vi "Beam_Max_Pos.vi"(1 "Picture Log":path, 5 "Search Step (mm)":dbl=1.0, 6 "Mode":T6, 7 "Starting Position":dbl[](array[numeric]) format="%.1f", 8 "Traverse line In":T1 {"Carrier_2 Q (l/min)" format="%#.2f"; "Row Duration (mins)" format="%#.1f"; "Row No" min=0; "Trace Gas Concentration (%)" min=0.0 format="%#_4f"; "Carrier_1 Q (l/min)" format="%#.2f"; "Tunnel Speed" format="%#.2f"; "Start X" format="%#.2f"; "Start Y" format="%#.2f"; "Start Z" format="%#.2f"; "End X" format="%#.2f"; "End Y" format="%#.2f"; "End Z" format="%#.2f"; "Averaging time (min)" min=0.0 format="%#.2f"}, 9 "Fixed Axis":T4, 10 "Beam Name":string) -> (0 "Power at Maxima":dbl, 2 "Status":T5, 3 "Beam maxima":dbl[](array[numeric]) format="%.1f", 4 "Message":string)   [LabVIEW 2016]
uses:
  Controls/User_Specific_mode.ctl
  Gen Trav/Multi_Run_Status.ctl
  Gen Trav/Route mapping/Axis.ctl
  Gen Trav/Traverse_cluster.ctl
  Gen Trav/Spacing.ctl
  Controls/Multi_run_mode.ctl
panel:
  out "Server copy Location":path
  out "vi reference":refnum<vi>
  in  "stop":bool
  out "Y":i32
  out "X":i32
  out "Array 2":dbl[](array[numeric]) format="%.4f"
  out "Measured Points":dbl[][](array[numeric]) format="%.2f"
  out "Current Value":dbl format="%.2f"
  out "Current Index":i32
  out "Array":i32[][](array[numeric])
  out "Light Power Measurement":dbl[][](graph)
  out "Found Maxima?":bool
  out "Present Position":dbl[](array[numeric])
  out "Profile":dbl[][](array[numeric]) format="%.2f"
  out "Log File":path
  # "X           Y            Z"
  # "Start"
  # "End"
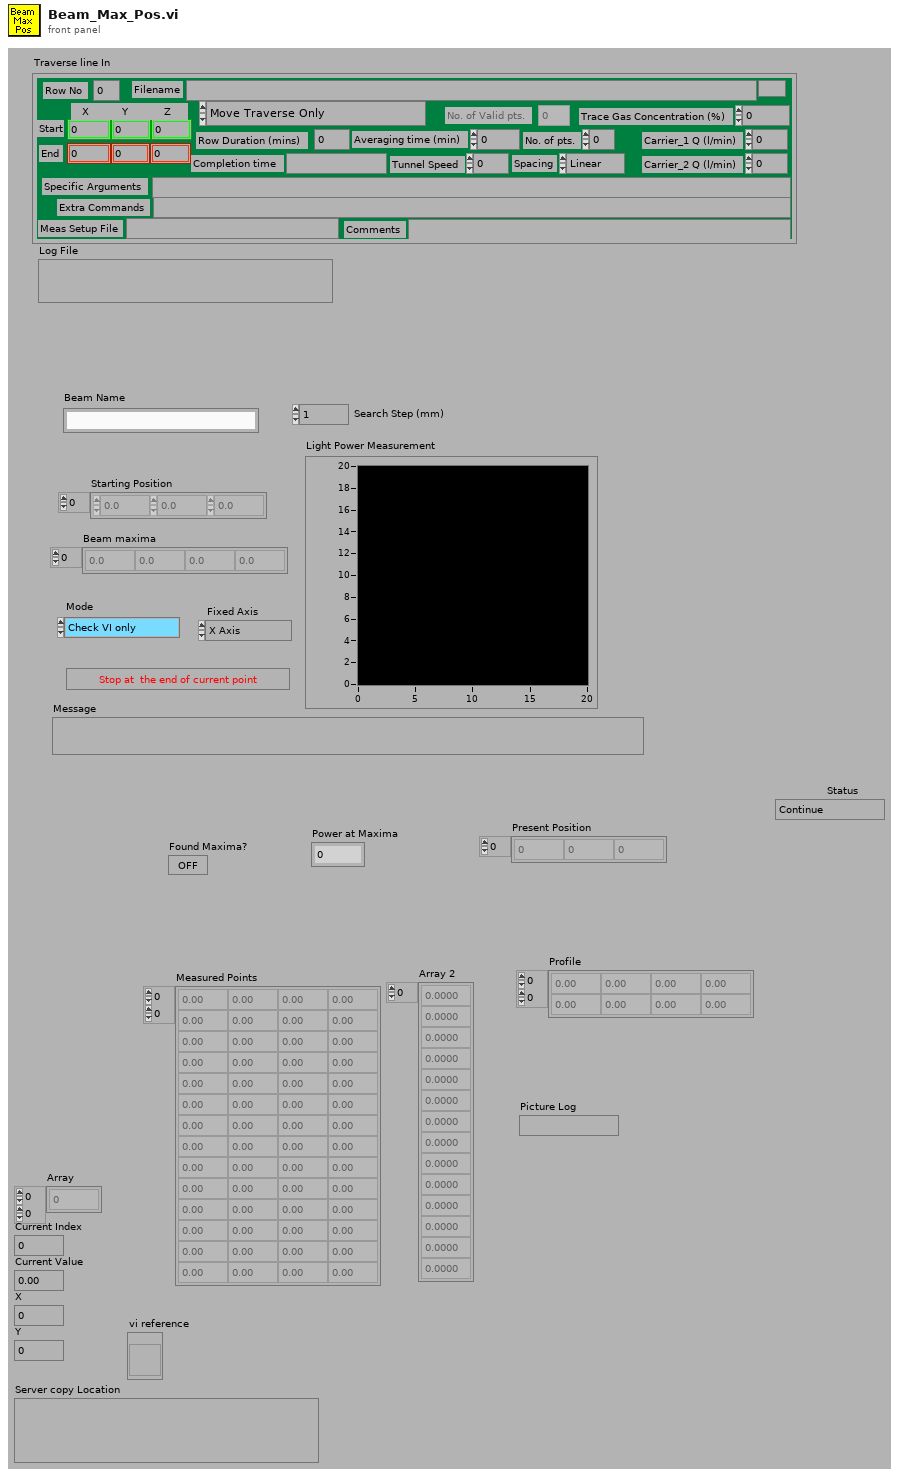
[diagram p1: front panel]
types:
  T1 = typedef "Traverse_cluster.ctl" = cluster{"Start X":sgl, "Start Y":sgl, "Start Z":sgl, "End X":sgl, "End Y":sgl, "End Z":sgl, "No. of pts.":i32, "Spacing":T2, "Filename":path, "Tunnel Speed":dbl, "Averaging time (min)":dbl, "Extra Commands":string, "Carrier_1 Q (l/min)":dbl, "Carrier_2 Q (l/min)":dbl, "Trace Gas Concentration (%)":dbl, "Specific Arguments":string, "Comments":string, "Row No":i32, "Row Type Selector":T3, "Completion time":string, "Row Duration (mins)":dbl, "No. of Valid pts.":i32, "Meas Setup File":string}
  T2 = typedef "Spacing.ctl" = enum16{"Linear", "Log", "Gauss", "Specified", "N/A"}
  T3 = typedef "Multi_run_mode.ctl" = enum16{"Move Traverse Only", "Set Tunnel Speed Only", "Set Source Only", "Set Measurement Conditions", "Single Measurement", "Vertical Profile", "Lateral Profile", "Longitudinal Profile", "Explore Volume", "Multi-Axis Profile", "Auto Calibrate", "Meas Fast FID Bkgnd", "Check Beam Power", "Scanning Valve Measurement", "Run VI Named:", "Set ADAM Ch", "Wait (minutes)", "Send Message", "Synchronize With:", "Fall Back to this Row", "Turn Off Row Repeating", "Blank Row", "Traverse 3D Volume"}
  T4 = typedef "Axis.ctl" = enum16{"X Axis", "X Axis -ve", "Y Axis", "Y Axis -ve", "Z Axis", "Z Axis -ve"}
  T5 = typedef "Multi_Run_Status.ctl" = enum16{"Continue", "Jump to Next Point", "Jump to Next Row", "Jump To Fall Back", "Terminate Run"}
  T6 = typedef "User_Specific_mode.ctl" = enum16{"Check VI only", "Run VI"}
  T7 = cluster{"Status":enum16{"Continue", "Jump to Next Point", "Jump to Next Row", "Jump To Fall Back", "Terminate Run"}, "Error Type":string, "Error Description":string}
  T8 = typedef "Status_Cluster.ctl" = cluster{"Status":T5, "Error Type":string, "Error Description":string}
  T9 = cluster{"second":i32, "minute":i32, "hour":i32, "day of month":i32, "month":i32, "year":i32, "day of week":i32, "day of year":i32, "is DST":i32}
  T10 = typedef "LVRectTypeDef.ctl" = cluster{"left":i16, "top":i16, "right":i16, "bottom":i16}
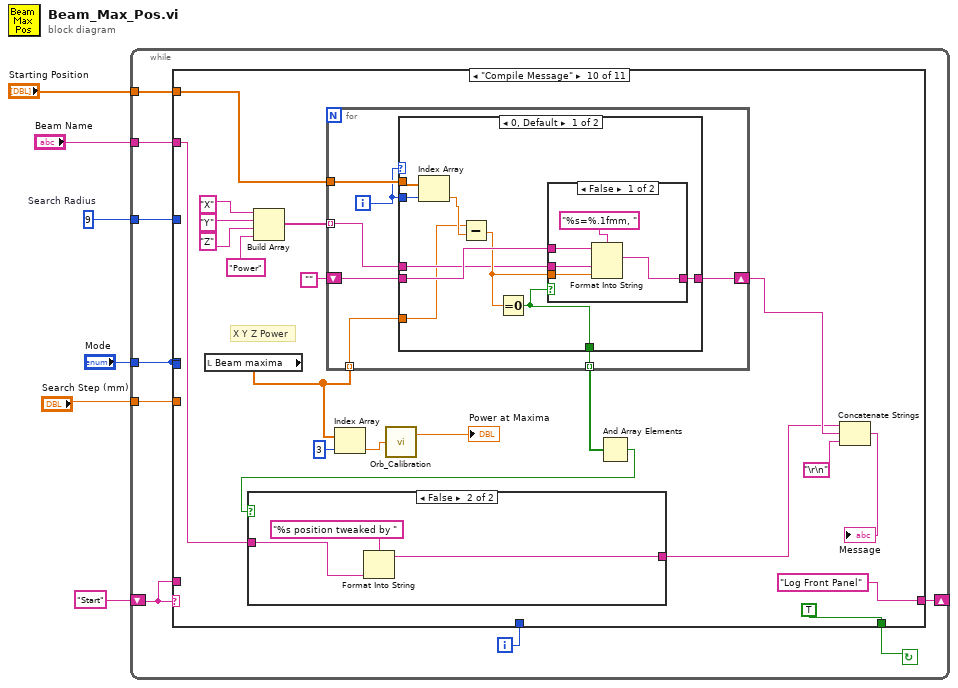
[diagram p0: block diagram]
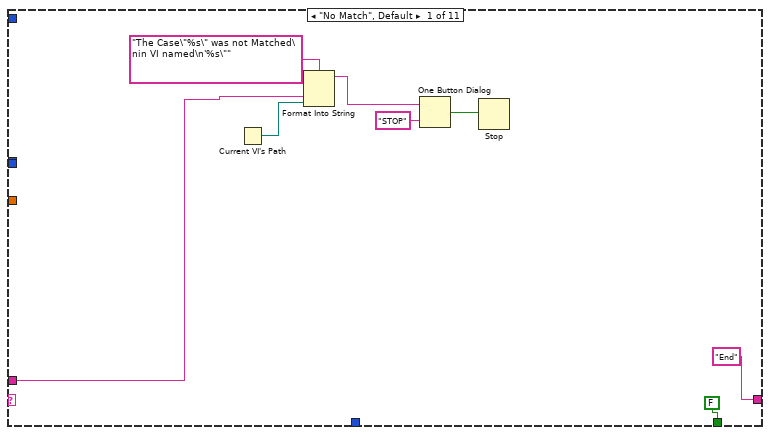
[diagram p2: hidden frame]
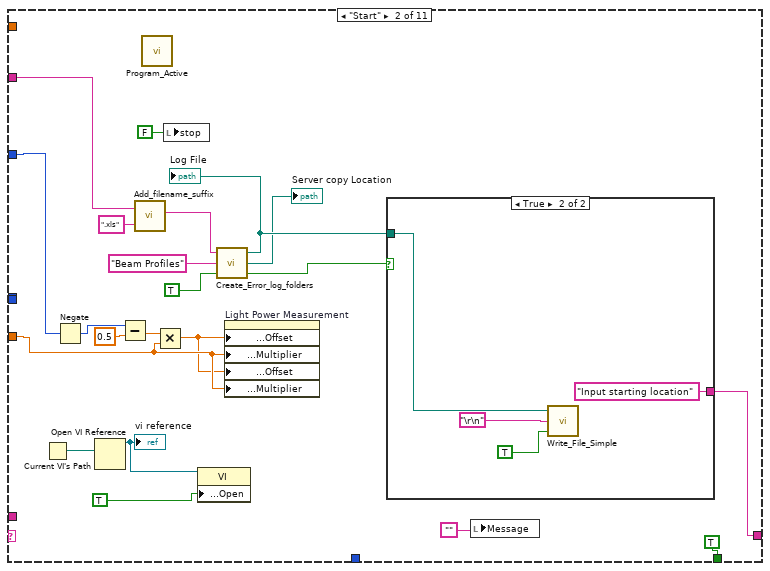
[diagram p3: hidden frame]
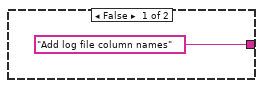
[diagram p4: hidden frame]
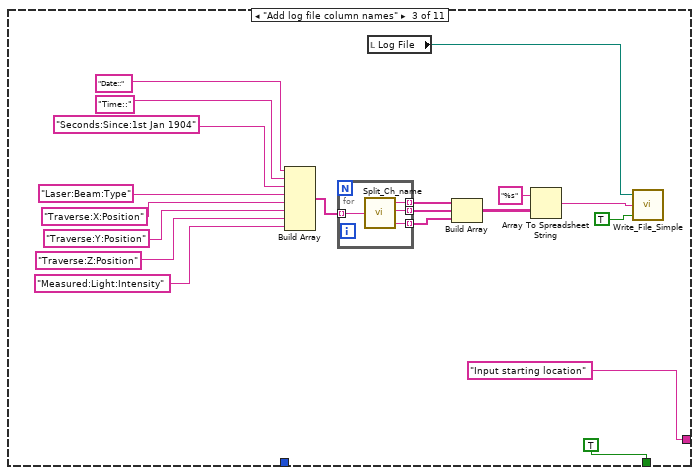
[diagram p5: hidden frame]
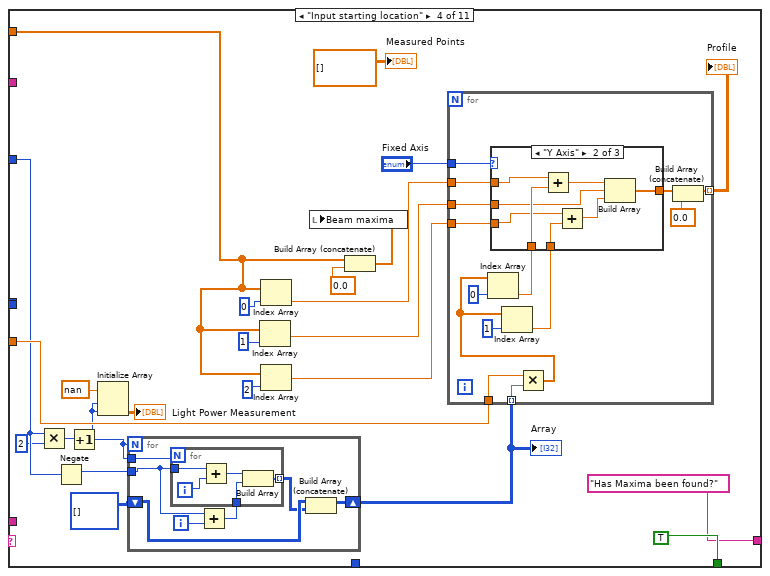
[diagram p6: hidden frame]
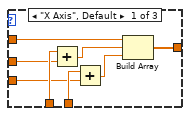
[diagram p7: hidden frame]
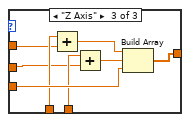
[diagram p8: hidden frame]
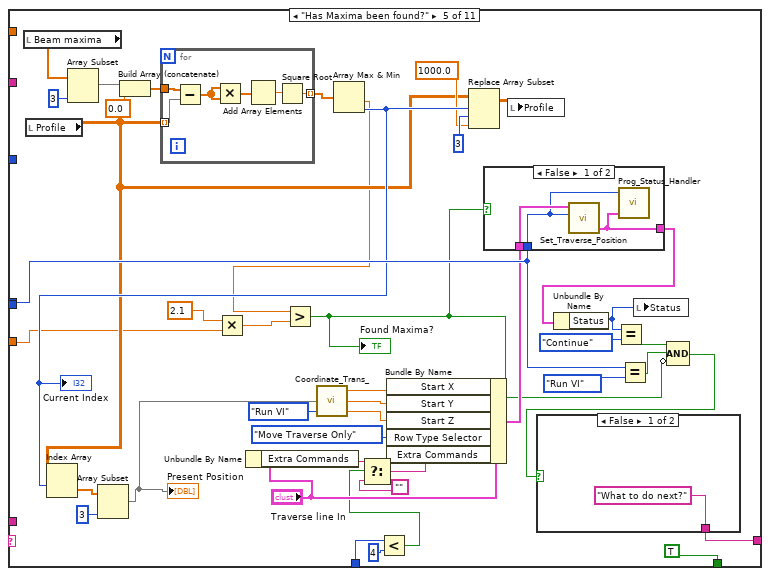
[diagram p9: hidden frame]
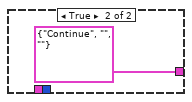
[diagram p10: hidden frame]
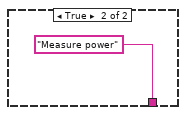
[diagram p11: hidden frame]
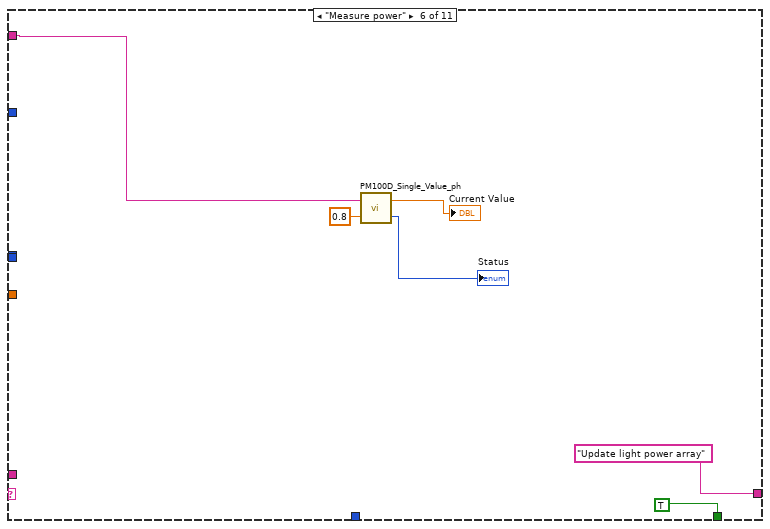
[diagram p12: hidden frame]
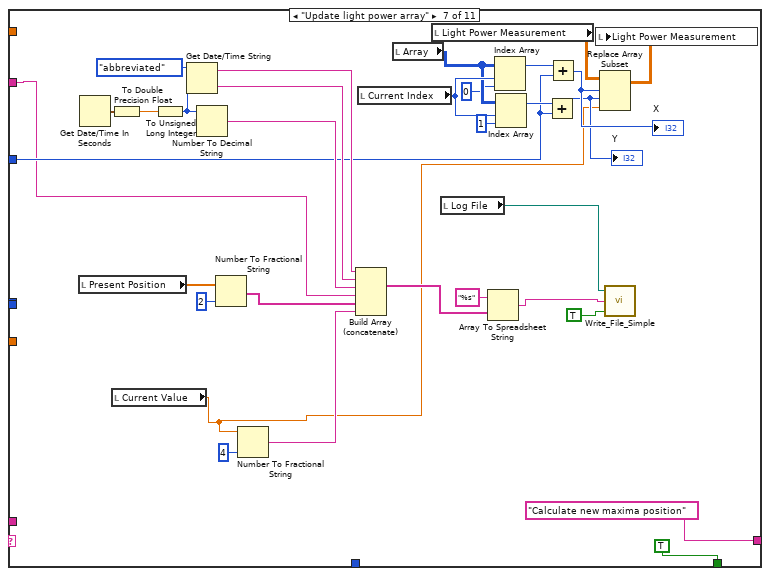
[diagram p13: hidden frame]
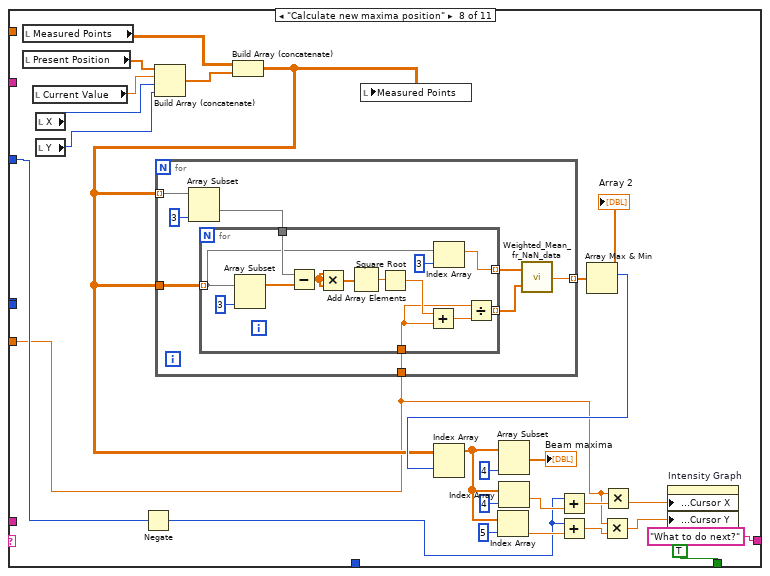
[diagram p14: hidden frame]
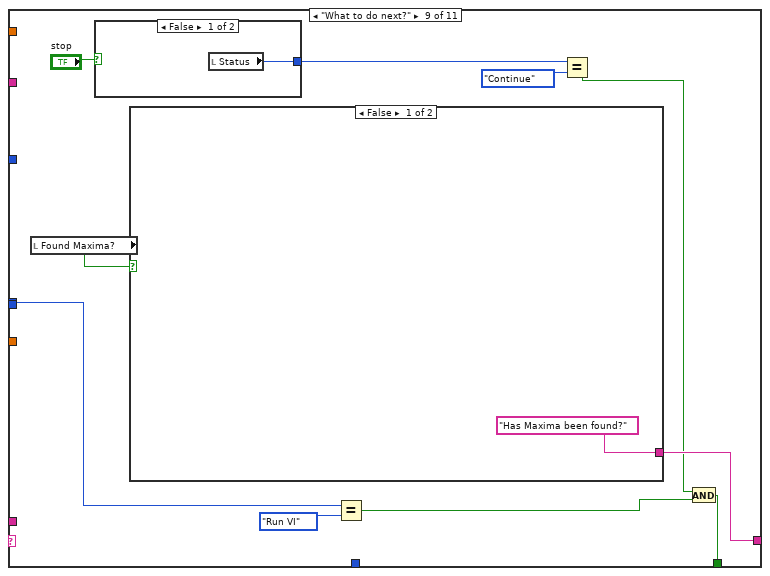
[diagram p15: hidden frame]
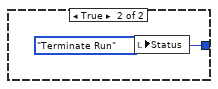
[diagram p16: hidden frame]
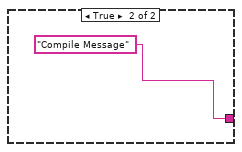
[diagram p17: hidden frame]
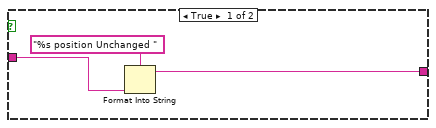
[diagram p18: hidden frame]
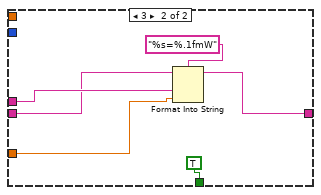
[diagram p20: hidden frame]
diagram:
  w5 = 9  # Search Radius
  n1 = while {
    tunnel: "Search Step (mm)" -> [w12]
    tunnel: "Mode" -> [w13]
    shift-left: "Start" -> [w7]
    shift-right: [w14] -> _
    tunnel: w5 -> [w11]
    tunnel: "Beam Name" -> [w10]
    tunnel: "Starting Position" -> [w9]
    i -> [w8]
    stop <- w15 continue-if-true
    n2 = case shown="\"Compile Message\"" w7 {
      tunnel: w13 -> [_ _ _ _ w184 _ _ _ w291 _ _]
      tunnel: [FALSE TRUE TRUE TRUE TRUE TRUE TRUE TRUE w285 TRUE FALSE] -> w15
      tunnel: ["End" w34 "Input starting location" "Has Maxima been found?" w163 "Update light power array" "Calculate new maxima position" "What to do next?" w288 "Log Front Panel" "End"] -> w14
      tunnel: w13 -> [_ _ _ _ _ _ _ _ _ _ _]
      tunnel: w12 -> [_ w33 _ w89 w165 _ _ w242 _ _ _]
      tunnel: w11 -> [_ w39 _ w81 _ _ w213 w246 _ _ _]
      tunnel: w10 -> [_ w37 _ _ _ w202 w211 _ _ w309 w359]
      tunnel: w9 -> [_ _ _ w74 _ _ _ _ _ w308 _]
      tunnel: w8 -> [_ _ _ _ w148 _ _ _ _ _ _]
      tunnel: w7 -> [w18 _ _ _ _ _ _ _ _ _ _]
      frame "No Match", Default {
        n3 = Current VI's Path() -> (path=w23:path)
        n4 = Format Into String(format string="The Case\"%s\" was not Matched\nin VI named\n'%s\"" ("Format String"), w18, w23) -> (resulting string=w20:string)  [unwired: 2 in, 1 out]
        n5 = One Button Dialog(message=w20, button name ("OK")="STOP") -> (true=w22:bool)
        n6 = Stop(stop? (T)=w22) -> ()
      }
      frame "Start" {
        n7 = Current VI's Path() -> (path=w28:path)
        n8 = Negate(x=w39) -> (-x=w30:i32)
        n9 = Open VI Reference(vi path=w28) -> (vi reference=w27:refnum<vi>)  [unwired: 1 in, 5 out]
        "vi reference" <- w27
        n10 = Subtract(x=w30, y=0.5) -> (x-y=w31:dbl)
        n11 = call "Add_filename_suffix.vi"("Filename"=w37, "Suffix to add"=".xls") -> ("Filename out"=w35:string)  [unwired: 3 out]
        n12 = call "Program_Active.vi"() -> ()  [unwired: 1 in]
        n13 = Multiply(x=w31, y=w33) -> (x*y=w32:dbl)
        n14 = local write "stop"(FALSE ("stop")) -> ()
        n15 = property class="VI"(reference=w27, "Front Panel Window:Open"=TRUE) -> ()  [unwired: 1 in, 2 out]
        n16 = call "Create_Error_log_folders.vi"("Per Day Log File?"=TRUE, "Log Folder"="Beam Profiles" ("Input Element"), "Log Filename"=w35) -> ("exists?"=w42:bool, "Server copy Location"=→"Server copy Location":path, "Local Log File"=w43:path)
        "Log File" <- w43
        n17 = property on="Light Power Measurement" class="IntGraph (strict)"("X Scale.Offset and Multiplier:Offset"=w32, "X Scale.Offset and Multiplier:Multiplier"=w33, "Y Scale.Offset and Multiplier:Offset"=w32, "Y Scale.Offset and Multiplier:Multiplier"=w33) -> ()  [unwired: 2 in, 2 out]
        n18 = case shown="True" w42 {
          tunnel: w43 -> [_ w46]
          tunnel: ["Add log file column names" "Input starting location"] -> w34
          frame False {
          }
          frame True {
            n19 = call "Write_File_Simple.vi"("append to file? (new file:F)"=TRUE, "character string"="\r\n", "file path"=w46) -> ()  [unwired: 2 out]
          }
        }
        n20 = local write "Message"("") -> ()
      }
      frame "Add log file column names" {
        n21 = Build Array("Date::", "Time::", "Seconds:Since:1st Jan 1904", "Laser:Beam:Type", "Traverse:X:Position", "Traverse:Y:Position", "Traverse:Z:Position", "Measured:Light:Intensity") -> (w62:string[])
        n22 = for {
          tunnel: w62 -> [w72] mode=indexing
          tunnel: [w71] -> w63 mode=indexing
          tunnel: [w70] -> w64 mode=indexing
          tunnel: [w69] -> w65 mode=indexing
          n23 = call "Split_Ch_name.vi"("Ch name"=w72) -> ("Top level"=w71:string, "Middle"=w70:string, "Low level"=w69:string)
        }
        n24 = local read "Log File"() -> (w50:path)
        n25 = Build Array(w63, w64, w65) -> (w60:string[][])
        n26 = Array To Spreadsheet String(array=w60, 3:"%s" ("format string")) -> (spreadsheet string=w51:string)  [unwired: 1 out]
        n27 = call "Write_File_Simple.vi"("append to file? (new file:F)"=TRUE, "character string"=w51, "file path"=w50) -> ()  [unwired: 2 out]
      }
      frame "Input starting location" {
        n28 = Multiply(x=w81, y=2) -> (x*y=w79:i32)
        n29 = Negate(x=w81) -> (-x=w82:i32)
        n30 = Increment(x=w79) -> (x+1=w78:i32)
        n31 = Initialize Array(nan, w78, w78) -> (→"Light Power Measurement":dbl[][])
        n32 = for {
          N: w78 -> [_]
          tunnel: w78 -> [w103]
          tunnel: w82 -> [w101]
          shift-right: [w97] -> w87
          shift-left: i32[][] [] -> [w99]
          i -> [w102]
          n33 = Add(x=w101, y=w102) -> (x+y=w100:i32)
          n34 = for {
            N: w103 -> [_]
            tunnel: w101 -> [w107]
            tunnel: w100 -> [w105]
            tunnel: [w104] -> w98 mode=indexing
            i -> [w108]
            n35 = Add(x=w107, y=w108) -> (x+y=w106:i32)
            n36 = Build Array(w106, w105) -> (w104:i32[])
          }
          n37 = Build Array (concatenate)(w99, w98) -> (w97:i32[][])
        }
        "Array" <- w87
        n38 = Index Array(array=w74, index=1 ("Index")) -> (element=w93:dbl)
        n39 = Index Array(array=w74, index=0 ("Index")) -> (element=w94:dbl)
        n40 = Index Array(array=w74, index=2 ("Index")) -> (element=w92:dbl)
        n41 = Build Array (concatenate)(w74, 0.0 ("Numeric")) -> (w90:dbl[])
        n42 = local write "Beam maxima"(w90) -> ()
        n43 = for {
          tunnel: w89 -> [w122]
          tunnel: w87 -> [w121] mode=indexing
          tunnel: "Fixed Axis" -> [w120]
          tunnel: w94 -> [w116]
          tunnel: w93 -> [w113]
          tunnel: w92 -> [w112]
          tunnel: [w110] -> w95 mode=indexing
          n44 = Multiply(x=w122, y=w121) -> (x*y=w117:dbl[])
          n45 = Index Array(array=w117, index=0 ("Index")) -> (element=w115:dbl)
          n46 = Index Array(array=w117, index=1 ("Index")) -> (element=w114:dbl)
          n47 = case shown="\"Y Axis\"" w120 {
            tunnel: w116 -> [w130 w137 w141]
            tunnel: w115 -> [w129 w135 w144]
            tunnel: w114 -> [w128 w134 w143]
            tunnel: w113 -> [w127 w131 w142]
            tunnel: w112 -> [w126 w133 w145]
            tunnel: [w123 w138 w146] -> w111
            frame "X Axis", Default {
              n48 = Add(x=w129, y=w127) -> (x+y=w125:dbl)
              n49 = Add(x=w128, y=w126) -> (x+y=w124:dbl)
              n50 = Build Array(w130, w125, w124) -> (w123:dbl[])
            }
            frame "Y Axis" {
              n51 = Add(x=w137, y=w135) -> (x+y=w136:dbl)
              n52 = Add(x=w133, y=w134) -> (x+y=w132:dbl)
              n53 = Build Array(w136, w131, w132) -> (w138:dbl[])
            }
            frame "Z Axis" {
              n54 = Add(x=w144, y=w141) -> (x+y=w140:dbl)
              n55 = Add(x=w143, y=w142) -> (x+y=w139:dbl)
              n56 = Build Array(w140, w139, w145) -> (w146:dbl[])
            }
          }
          n57 = Build Array (concatenate)(w111, 0.0 ("Input Element")) -> (w110:dbl[])
        }
        "Profile" <- w95
        "Measured Points" <- dbl[][] [] ("Measured Points")
      }
      frame "Has Maxima been found?" {
        n58 = local read "Beam maxima"() -> (w181:dbl[])
        n59 = local read "Profile"() -> (w171:dbl[][])
        n60 = Array Subset(array=w181, length=3 ("Array Length")) -> (w178:dbl[])  [unwired: 1 in]
        n61 = Build Array (concatenate)(w178, 0.0 ("Input Element")) -> (w177:dbl[])
        n62 = for {
          tunnel: w171 -> [w200] mode=indexing
          tunnel: w177 -> [w199]
          tunnel: [w195] -> w179 mode=indexing
          n63 = Subtract(x=w199, y=w200) -> (x-y=w197:dbl[])
          n64 = Multiply(x=w197, y=w197) -> (x*y=w196:dbl[])
          n65 = Add Array Elements(numeric array=w196) -> (sum=w198:dbl)
          n66 = Square Root(x=w198) -> (sqrt(x)=w195:dbl)
        }
        n67 = Multiply(x=2.1, y=w165) -> (x*y=w168:dbl)
        n68 = Unbundle By Name("Traverse line In") -> ("Extra Commands"=w160:string)
        n69 = Array Max & Min(array=w179) -> (min value=w169:dbl, min index (indices)=w175:i32)  [unwired: 2 out]
        "Current Index" <- w175
        n70 = Index Array(array=w171, index (row)=w175) -> (element=w151:dbl[])  [unwired: 1 in]
        n71 = Array Subset(array=w151, length=3) -> (w150:dbl[])  [unwired: 1 in]
        "Present Position" <- w150
        n72 = Greater?(x=w169, y=w168) -> (0:w155:bool)
        "Found Maxima?" <- w155
        n73 = call "Coordinate_Trans_.vi"("Simulate/Run"=User_Specific_mode."Run VI", "Input Position"=w150) -> ("Z"=w154:sgl, "Y"=w153:sgl, "X"=w152:sgl)  [unwired: 1 in]
        n74 = Less?(x=w148, y=4) -> (x < y?=w158:bool)
        n75 = Select(t=w160, s=w158, f="") -> (s? t:f=w156:string)
        n76 = Bundle By Name(cluster="Traverse line In", "Start X"=w152, "Start Y"=w153, "Start Z"=w154, "Row Type Selector"=Multi_run_mode."Move Traverse Only", "Extra Commands"=w156) -> (w164:T1)
        n77 = Replace Array Subset(array=w171, new element=1000.0 ("Element Data"), index (row)=w175, index (col)=3 ("Index")) -> (w172:dbl[][])
        n78 = case shown="False" w155 {
          tunnel: [w190 T7 {"Status"=enum."Continue", "Error Type"="", "Error Description"=""} ("Status Cluster")] -> w186
          tunnel: w184 -> [w189 _]
          tunnel: w164 -> [w191 _]
          frame False {
            n79 = call "Set_Traverse_Position.vi"("Simulate/Run"=w189, "Traverse line"=w191) -> ("Status Cluster"=w190:T8)  [unwired: 4 in]
            n80 = call "Prog_Status_Handler.vi"("Status Cluster"=w190, "Simulate/Run"=w189) -> ()  [unwired: 2 out]
          }
          frame True {
          }
        }
        n81 = local write "Profile"(w172) -> ()
        n82 = Unbundle By Name(w186) -> ("Status"=w182:T5)
        n83 = Equal?(x=w182, y=Multi_Run_Status."Continue" ("Status")) -> (x = y?=w167:bool)
        n84 = Equal?(x=w184, y=User_Specific_mode."Run VI" ("Mode")) -> (x = y?=w166:bool)
        n85 = local write "Status"(w182) -> ()
        n86 = Compound Arithmetic op=AND(w167, w166, invert w155) -> (w162:bool)
        n87 = case shown="False" w162 {
          tunnel: ["What to do next?" "Measure power"] -> w163
          frame False {
          }
          frame True {
          }
        }
      }
      frame "Measure power" {
        n88 = call "PM100D_Single_Value_ph.vi"("Averaging Period (s)"=0.8, "Beam Name"=w202) -> ("Status"=→"Status":T5, "Light Power mW"=→"Current Value":dbl)
      }
      frame "Update light power array" {
        n89 = local read "Present Position"() -> (w225:dbl[])
        n90 = Get Date/Time In Seconds() -> (seconds since 1Jan1904=w214:timestamp)
        n91 = To Double Precision Float(number=w214) -> (double precision float=w235:dbl)
        n92 = local read "Current Value"() -> (w207:dbl)
        n93 = To Unsigned Long Integer(number=w235) -> (unsigned 32bit integer=w234:u32)
        n94 = Get Date/Time String(date format (0)=enum16{"short", "long", "abbreviated"}."abbreviated", seconds (now)=w234) -> (date string=w233:string, time string=w232:string)  [unwired: 1 out]
        n95 = Number To Decimal String(number=w234) -> (decimal integer string=w231:string)  [unwired: 1 out]
        n96 = Number To Fractional String(number=w225, precision (6)=i16 2) -> (F-format string=w226:string[])  [unwired: 2 out]
        n97 = Number To Fractional String(number=w207, precision (6)=i16 4) -> (F-format string=w227:string)  [unwired: 2 out]
        n98 = Build Array (concatenate)(w233, w232, w231, w211, w226, w227) -> (w230:string[])
        n99 = local read "Current Index"() -> (w224:i32)
        n100 = local read "Array"() -> (w223:i32[][])
        n101 = local read "Light Power Measurement"() -> (w220:dbl[][])
        n102 = local read "Log File"() -> (w208:path)
        n103 = Array To Spreadsheet String(array=w230, 3:"%s" ("format string")) -> (spreadsheet string=w209:string)  [unwired: 1 out]
        n104 = Index Array(array=w223, index (row)=w224, index (col)=0 ("Index")) -> (element=w217:i32)
        n105 = Index Array(array=w223, index (row)=w224, index (col)=1 ("Index")) -> (element=w218:i32)
        n106 = Add(x=w218, y=w213) -> (x+y=w215:i32)
        "Y" <- w215
        n107 = Add(x=w217, y=w213) -> (x+y=w216:i32)
        "X" <- w216
        n108 = Replace Array Subset(array=w220, new element=w207, index (row)=w216, index (col)=w215) -> (w219:dbl[][])
        n109 = local write "Light Power Measurement"(w219) -> ()
        n110 = call "Write_File_Simple.vi"("append to file? (new file:F)"=TRUE, "character string"=w209, "file path"=w208) -> ()  [unwired: 2 out]
      }
      frame "Calculate new maxima position" {
        n111 = local read "Measured Points"() -> (w262:dbl[][])
        n112 = local read "Present Position"() -> (w261:dbl[])
        n113 = local read "Current Value"() -> (w260:dbl)
        n114 = local read "X"() -> (w255:i32)
        n115 = local read "Y"() -> (w254:i32)
        n116 = Negate(x=w246) -> (-x=w244:i32)
        n117 = Build Array (concatenate)(w261, w260, w255, w254) -> (w259:dbl[])
        n118 = Build Array (concatenate)(w262, w259) -> (w256:dbl[][])
        n119 = for {
          tunnel: w256 -> [w271] mode=indexing
          tunnel: w256 -> [w269]
          tunnel: w242 -> [w267]
          tunnel: [w264] -> w258 mode=indexing
          n120 = Array Subset(array=w271, length=3 ("Array Length")) -> (w268:dbl[])  [unwired: 1 in]
          n121 = for {
            tunnel: w269 -> [w278] mode=indexing
            tunnel: w268 -> [w283]
            tunnel: w267 -> [w273]
            tunnel: [w275] -> w265 mode=indexing
            tunnel: [w272] -> w266 mode=indexing
            n122 = Array Subset(array=w278, length=3 ("Array Length")) -> (w282:dbl[])  [unwired: 1 in]
            n123 = Subtract(x=w283, y=w282) -> (x-y=w279:dbl[])
            n124 = Multiply(x=w279, y=w279) -> (x*y=w280:dbl[])
            n125 = Add Array Elements(numeric array=w280) -> (sum=w281:dbl)
            n126 = Square Root(x=w281) -> (sqrt(x)=w276:dbl)
            n127 = Add(x=w276, y=w273) -> (x+y=w274:dbl)
            n128 = Index Array(array=w278, index=3 ("Index")) -> (element=w272:dbl)
            n129 = Divide(x=w273, y=w274) -> (x/y=w275:dbl)
          }
          n130 = call "Weighted_Mean_fr_NaN_data.vi"("Weighting"=w265, "Data"=w266) -> ("Mean value"=w264:dbl)
        }
        "Array 2" <- w258
        n131 = local write "Measured Points"(w256) -> ()
        n132 = Array Max & Min(array=w258) -> (max index (indices)=w257:i32)  [unwired: 3 out]
        n133 = Index Array(array=w256, index (row)=w257) -> (element=w249:dbl[])  [unwired: 1 in]
        n134 = Index Array(array=w249, index=5 ("Index")) -> (element=w247:dbl)
        n135 = Array Subset(array=w249, length=4 ("Array Length")) -> (→"Beam maxima":dbl[])  [unwired: 1 in]
        n136 = Index Array(array=w249, index=4 ("Index")) -> (element=w248:dbl)
        n137 = Add(x=w244, y=w248) -> (x+y=w243:dbl)
        n138 = Add(x=w244, y=w247) -> (x+y=w241:dbl)
        n139 = Multiply(x=w242, y=w241) -> (x*y=w240:dbl)
        n140 = Multiply(x=w242, y=w243) -> (x*y=w239:dbl)
        n141 = property on="Intensity Graph" class="IntGraph (strict)"("Cursor.Cursor Position:Cursor X"=w239, "Cursor.Cursor Position:Cursor Y"=w240) -> ()  [unwired: 2 in, 2 out]
      }
      frame "What to do next?" {
        n142 = local read "Found Maxima?"() -> (w293:bool)
        n143 = case shown="False" "stop" {
          tunnel: [w295 w296] -> w289
          frame False {
            n144 = local read "Status"() -> (w295:T5)
          }
          frame True {
            w296 = Multi_Run_Status."Terminate Run" ("Status")
            n145 = local write "Status"(w296) -> ()
          }
        }
        n146 = case shown="False" w293 {
          tunnel: ["Has Maxima been found?" "Compile Message"] -> w288
          frame False {
          }
          frame True {
          }
        }
        n147 = Equal?(x=w291, y=User_Specific_mode."Run VI" ("Mode")) -> (x = y?=w287:bool)
        n148 = Equal?(x=w289, y=Multi_Run_Status."Continue" ("Status")) -> (x = y?=w286:bool)
        n149 = And(x=w286, y=w287) -> (x .and. y?=w285:bool)
      }
      frame "Compile Message" {
        # "X Y Z Power"
        n150 = local read "Beam maxima"() -> (w307:dbl[])
        n151 = Build Array("X", "Y", "Z", "Power" ("Input Element")) -> (w314:string[])
        n152 = for {
          tunnel: w307 -> [w331] mode=indexing
          shift-right: [w329] -> w313
          shift-left: "" -> [w330]
          tunnel: w314 -> [w328] mode=indexing
          tunnel: [w327] -> w310 mode=indexing
          tunnel: w308 -> [w326]
          i -> [w325]
          n153 = case shown="0, Default" w325 {
            tunnel: w331 -> [w332 w350]
            tunnel: w330 -> [w340 w348]
            tunnel: [w339 w347] -> w329
            tunnel: w328 -> [w333 w352]
            tunnel: [w337 TRUE] -> w327
            tunnel: w326 -> [w336 _]
            tunnel: w325 -> [w335 _]
            frame 0, Default {
              n154 = Index Array(array=w336, index=w335) -> (element=w334:dbl)
              n155 = Subtract(x=w332, y=w334) -> (x-y=w338:dbl)
              n156 = Equal To 0?(x=w338) -> (x = 0?=w337:bool)
              n157 = case shown="False" w337 {
                tunnel: w340 -> [w345 w346]
                tunnel: [w344 w346] -> w339
                tunnel: w333 -> [w343 _]
                tunnel: w338 -> [w341 _]
                frame False {
                  n158 = Format Into String(format string="%s=%.1fmm, " ("Format String"), initial string=w345, w343, w341) -> (resulting string=w344:string)  [unwired: 1 in, 1 out]
                }
                frame True {
                }
              }
            }
            frame 3 {
              n159 = Format Into String(format string="%s=%.1fmW" ("Format String"), initial string=w348, w352, w350) -> (resulting string=w347:string)  [unwired: 1 in, 1 out]
            }
          }
        }
        n160 = Index Array(array=w307, index=3) -> (element=w305:dbl)
        n161 = call "Orb_Calibration.vi"("Voltage"=w305) -> ("Normalised Voltage"=→"Power at Maxima":dbl)  [unwired: 1 out]
        n162 = And Array Elements(Boolean array=w310) -> (logical AND=w302:bool)
        n163 = case shown="False" w302 {
          tunnel: [w320 w323] -> w312
          tunnel: w309 -> [w319 w322]
          frame True {
            n164 = Format Into String(format string="%s position Unchanged " ("Format String"), w319) -> (resulting string=w320:string)  [unwired: 2 in, 1 out]
          }
          frame False {
            n165 = Format Into String(format string="%s position tweaked by " ("Format String"), w322) -> (resulting string=w323:string)  [unwired: 2 in, 1 out]
          }
        }
        n166 = Concatenate Strings(w312, w313, "\r\n") -> (→"Message":string)
      }
      frame "Log Front Panel" {
        w366 = 8 ("image depth")
        n167 = local read "Server copy Location"() -> (w353:path)
        n168 = Empty String/Path?(string/path="Picture Log") -> (empty?=w364:bool)
        n169 = local read "vi reference"() -> (w357:refnum<vi>)
        n170 = local read "Log File"() -> (w354:path)
        n171 = case shown="True" w364 {
          tunnel: [w375 w378] -> w363
          tunnel: "Picture Log" -> [w375 _]
          frame False {
          }
          frame True {
            n172 = Get Date/Time In Seconds() -> (seconds since 1Jan1904=w376:timestamp)
            n173 = call <vilib>:"LV70TimeStampToDateRec.vi"("time stamp"=w376) -> ("date time rec"=w381:T9)
            n174 = Unbundle By Name(w381) -> ("day of month"=w384:i32, "hour"=w383:i32, "minute"=w382:i32)
            n175 = call "Create_Error_log_folders.vi"("Log Folder"="Beam_Max_Pos" ("name or relative path"), "Log Filename"="test") -> ("Server copy Location"=w377:path)  [unwired: 1 in, 2 out]
            n176 = Strip Path(path=w377) -> (stripped path=w380:path)  [unwired: 1 out]
            n177 = Format Into String(format string="Day%02d_Time%02d-%02d", w384, w383, w382) -> (resulting string=w379:string)  [unwired: 2 in, 1 out]
            n178 = Build Path(base path=w380, name or relative path=w379) -> (appended path=w378:path)
          }
        }
        n179 = Close Reference(reference=w357) -> ()  [unwired: 1 in, 1 out]
        n180 = call "Updated_File_Copy.vi"("Target Path"=w353, "Source Path"=w354) -> ()  [unwired: 2 out]
        n181 = Current VI's Path() -> (path=w374:path)
        n182 = Open VI Reference(vi path=w374) -> (vi reference=w373:refnum<vi>, error out=w372:errorcluster)  [unwired: 1 in, 4 out]
        n183 = invoke class="VI" method="FP.Old Get Image"(reference=w373, error in=w372, "visible area only"=TRUE, "image depth"=w366) -> (error out=w370:errorcluster, "image"=w369:u8[], "colors"=w367:u32[], "bounds"=w368:T10)  [unwired: 4 in, 4 out]
        n184 = Concatenate Strings(w359, ".png" ("string")) -> (w360:string)
        n185 = Build Path(base path=w363, name or relative path=w360) -> (appended path=w356:path)
        n186 = call "Create_directory_path.vi"("Path name"=w356) -> ("Path name Out"=w355:path)  [unwired: 2 in, 1 out]
        n187 = call <vilib>:"Write PNG File(6_1).vi"("color table"=w367, "depth"=w366, "error in (no error)"=w370, "flattened image data"=w369, "rect"=w368, "path to PNG file"=w355) -> ()  [unwired: 6 out]
      }
    }
  }
